vi "setSerializedData.vi"(0 "reference":refnum<class "CallEdge.lvclass">, 1 "startNode":refnum<class "AbstractNode.lvclass">, 2 "endNode":refnum<class "AbstractNode.lvclass">, 3 "xmlOut":string, 5 "error in (no error)":errorcluster) -> (14 "reference out":refnum<class "CallEdge.lvclass">, 19 "error out":errorcluster)   [LabVIEW 2014, in "CallEdge.lvclass"]
doc: "setSerializedData"
uses:
  <resource>/Framework/Providers/Open_GDS/UML/CallEdge_class/CallEdge.lvclass
  <resource>/Framework/Providers/Open_GDS/UML/AbstractNode_class/AbstractNode.lvclass
  <resource>/Framework/Providers/Open_GDS/UML/General/Point/Point Point2D.ctl
  <resource>/Framework/Providers/Open_GDS/UML/LineStyle_class/LineStyleType.ctl
  <resource>/Framework/Providers/Open_GDS/UML/ArrowHead_class/ArrowHeadType.ctl
  <resource>/Framework/Providers/Open_GDS/UML/LineStyle_class/LineStyle.lvclass
  <resource>/Framework/Providers/Open_GDS/UML/ArrowHead_class/ArrowHead.lvclass
  <resource>/Framework/Providers/Open_GDS/UML/SegmentedLineEdge_class/SegmentedLineEdge.lvclass
  <resource>/Framework/Providers/Open_GDS/UML/AbstractEdge_class/AbstractEdge.lvclass
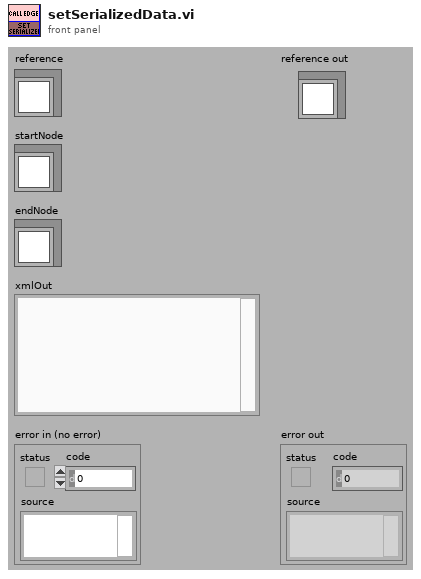
[diagram p1: front panel]
types:
  T1 = typedef "Point Point2D.ctl" = cluster{"x":dbl, "y":dbl}
  T2 = cluster{"Base class":cluster{"Base class":cluster{"Base class":cluster{"start":refnum<k1>, "end":refnum<k1>}}, "lineStyle":refnum<k1>, "startArrowHead":refnum<k1>, "endArrowHead":refnum<k1>, "startLabel":string, "midLabel":string, "endLabel":string, "MidLabelOffset":T1, "SplitWire":bool}, "signal":bool}
  T3 = typedef "LineStyle.lvclass/LineStyleType.ctl" = enum16{"SOLID", "DOTTED"}
  T4 = typedef "ArrowHead.lvclass/ArrowHeadType.ctl" = enum16{"NONE", "TRIANGLE", "BLACK_TRIANGLE", "V", "HALF_V", "DIAMOND", "BLACK_DIAMOND"}
  T5 = cluster{"Attributes":cluster{"Base class":cluster{"Base class":cluster{"Base class":cluster{"start":refnum<k1>, "end":refnum<k1>}}, "lineStyle":refnum<k1>, "startArrowHead":refnum<k1>, "endArrowHead":refnum<k1>, "startLabel":string, "midLabel":string, "endLabel":string, "MidLabelOffset":T1, "SplitWire":bool}, "signal":bool}, string, string, string}
  T6 = typedef "CallEdge.lvclass/ObjectAttributes.ctl" = cluster{"signal":bool}
  T7 = typedef "SegmentedLineEdge.lvclass/ObjectAttributes.ctl" = cluster{"lineStyle":refnum<class "LineStyle.lvclass">, "startArrowHead":refnum<class "ArrowHead.lvclass">, "endArrowHead":refnum<class "ArrowHead.lvclass">, "startLabel":string, "midLabel":string, "endLabel":string, "MidLabelOffset":T1, "SplitWire":bool}
  T8 = typedef "AbstractEdge.lvclass/ObjectAttributes.ctl" = cluster{"start":refnum<class "AbstractNode.lvclass">, "end":refnum<class "AbstractNode.lvclass">}
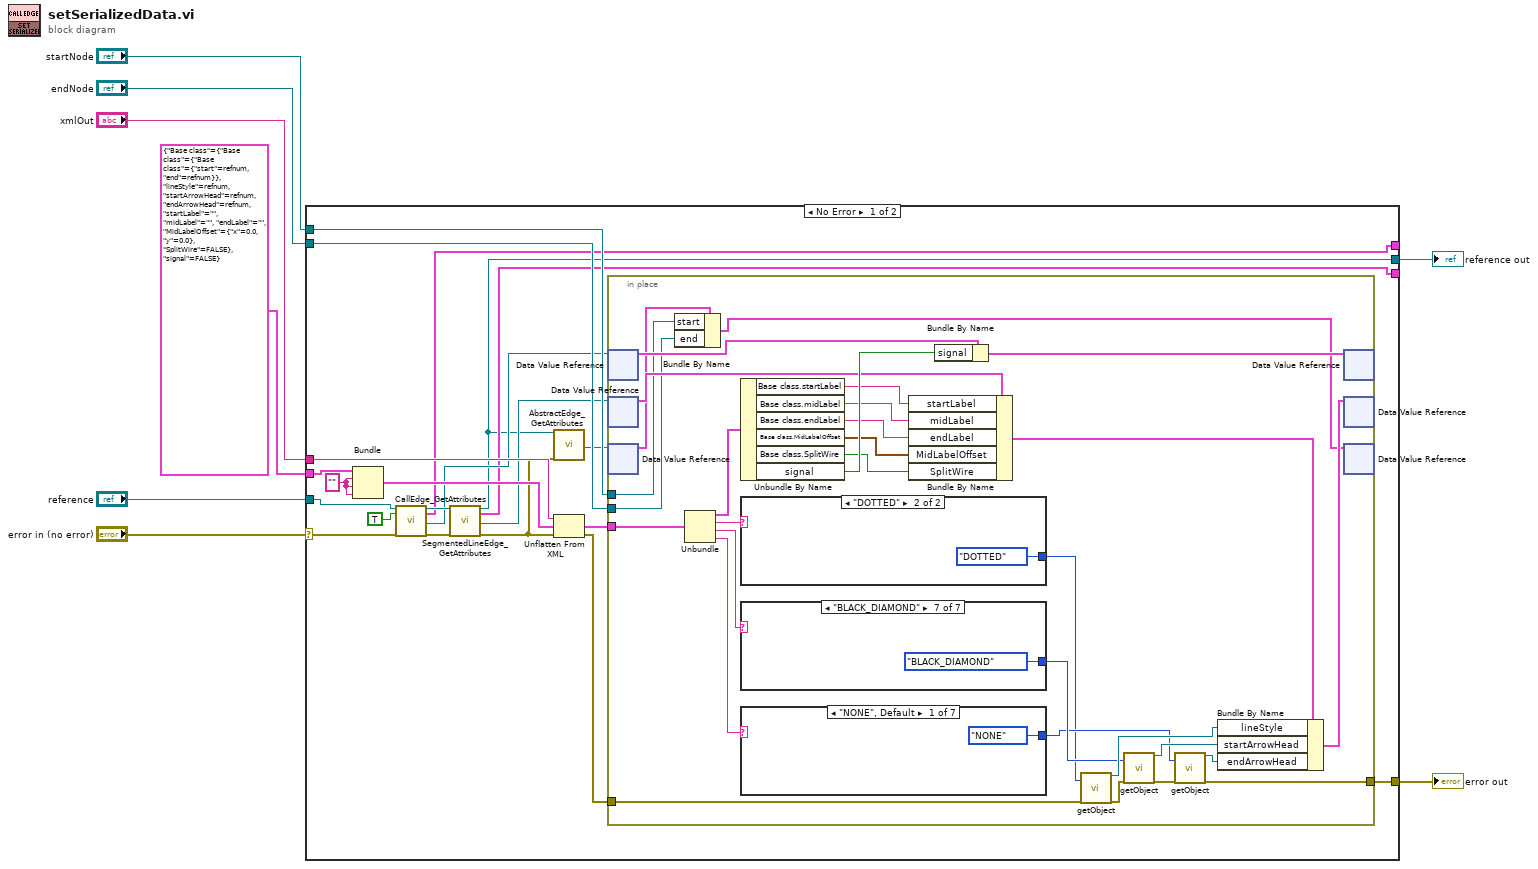
[diagram p0: block diagram]
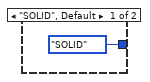
[diagram p2: hidden frame]
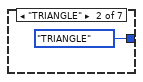
[diagram p3: hidden frame]
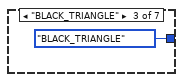
[diagram p4: hidden frame]
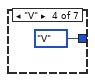
[diagram p5: hidden frame]
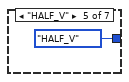
[diagram p6: hidden frame]
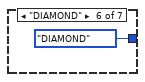
[diagram p7: hidden frame]
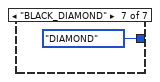
[diagram p8: hidden frame]
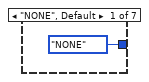
[diagram p9: hidden frame]
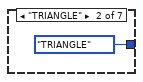
[diagram p10: hidden frame]
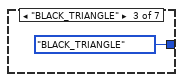
[diagram p11: hidden frame]
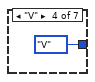
[diagram p12: hidden frame]
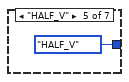
[diagram p13: hidden frame]
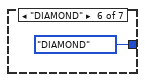
[diagram p14: hidden frame]
diagram:
  n1 = case shown="No Error" "error in (no error)" {
    selector: "error in (no error)" -> [w28 w76]
    tunnel: "reference" -> [w29 w77]
    tunnel: [w11 w77] -> w6
    tunnel: [w27 w76] -> w5
    tunnel: "xmlOut" -> [w18 _]
    tunnel: "startNode" -> [w26 _]
    tunnel: "endNode" -> [w25 _]
    tunnel: T2 {"Base class"={"Base class"={"Base class"={"start"=refnum, "end"=refnum}}, "lineStyle"=refnum, "startArrowHead"=refnum, "endArrowHead"=refnum, "startLabel"="", "midLabel"="", "endLabel"="", "MidLabelOffset"={"x"=0.0, "y"=0.0}, "SplitWire"=FALSE}, "signal"=FALSE} ("Attributes") -> [w23 _]
    tunnel: [w13 _] -> _
    tunnel: [w12 _] -> _
    frame No Error {
      w24 = ""
      n2 = Bundle("Attributes"=w23, w24, w24, w24) -> (w16:T5)  [unwired: 1 out]
      n3 = call <resource>:"CallEdge_GetAttributes.vi"("reference in"=w29, "OnlyGetDvrReference(False)"=TRUE, "error in (no error)"=w28) -> ("reference out"=w21:refnum<class "CallEdge.lvclass">, "Data"=w13:T6, "DataRef"=w15:refnum<data-value>, "error out"=w20:errorcluster)  [unwired: 13 in]
      n4 = call <resource>:"SegmentedLineEdge_GetAttributes.vi"("reference in"=w21, "error in (no error)"=w20) -> ("reference out"=w11:refnum<class "CallEdge.lvclass">, "Data"=w12:T7, "DataRef"=w14:refnum<data-value>, "error out"=w10:errorcluster)  [unwired: 14 in]
      n5 = call <resource>:"AbstractEdge_GetAttributes.vi"("reference in"=w11, "error in (no error)"=w10) -> ("DataRef"=w9:refnum<data-value>)  [unwired: 14 in, 3 out]
      n6 = Unflatten From XML(xml string=w18, type=w16, error in (no error)=w10) -> (value=w19:T5, error out=w17:errorcluster)
      n7 = in-place {
        in-place-border: [w54] -> w27
        in-place-border: w26 -> [w38]
        in-place-border: w25 -> [w37]
        in-place-border: w19 -> [w50]
        in-place-border: w17 -> [w49]
        n8 = in-place-dvr #1(w15) -> (w41:T6)  [unwired: 1 out]
        n9 = in-place-dvr #2(w14) -> (w39:T7)  [unwired: 1 out]
        n10 = in-place-dvr #3(w9) -> (w34:T8)  [unwired: 1 out]
        n11 = Bundle By Name(cluster=w34, "start"=w38, "end"=w37) -> (w33:T8)
        n12 = Unbundle(w50) -> ("Attributes"=w42:T2, w32:string, w31:string, w30:string)
        n13 = Unbundle By Name(w42) -> ("Base class.startLabel"=w43:string, "Base class.midLabel"=w44:string, "Base class.endLabel"=w45:string, "Base class.MidLabelOffset"=w46:T1, "Base class.SplitWire"=w47:bool, "signal"=w48:bool)
        n14 = case shown="\"DOTTED\"" w32 {
          tunnel: [LineStyleType."SOLID" ("lineStyle") LineStyleType."DOTTED" ("lineStyle")] -> w51
          frame "SOLID", Default {
          }
          frame "DOTTED" {
          }
        }
        n15 = case shown="\"BLACK_DIAMOND\"" w31 {
          tunnel: [ArrowHeadType."NONE" ("arrowHead") ArrowHeadType."TRIANGLE" ("arrowHead") ArrowHeadType."BLACK_TRIANGLE" ("arrowHead") ArrowHeadType."V" ("arrowHead") ArrowHeadType."HALF_V" ("arrowHead") ArrowHeadType."DIAMOND" ("arrowHead") ArrowHeadType."BLACK_DIAMOND" ("arrowHead")] -> w53
          frame "NONE", Default {
          }
          frame "TRIANGLE" {
          }
          frame "BLACK_TRIANGLE" {
          }
          frame "V" {
          }
          frame "HALF_V" {
          }
          frame "DIAMOND" {
          }
          frame "BLACK_DIAMOND" {
          }
        }
        n16 = case shown="\"NONE\", Default" w30 {
          tunnel: [ArrowHeadType."NONE" ("arrowHead") ArrowHeadType."TRIANGLE" ("arrowHead") ArrowHeadType."BLACK_TRIANGLE" ("arrowHead") ArrowHeadType."V" ("arrowHead") ArrowHeadType."HALF_V" ("arrowHead") ArrowHeadType."DIAMOND" ("arrowHead") ArrowHeadType."DIAMOND" ("arrowHead")] -> w52
          frame "NONE", Default {
          }
          frame "TRIANGLE" {
          }
          frame "BLACK_TRIANGLE" {
          }
          frame "V" {
          }
          frame "HALF_V" {
          }
          frame "DIAMOND" {
          }
          frame "BLACK_DIAMOND" {
          }
        }
        n17 = Bundle By Name(cluster=w39, "startLabel"=w43, "midLabel"=w44, "endLabel"=w45, "MidLabelOffset"=w46, "SplitWire"=w47) -> (w36:T7)
        n18 = Bundle By Name(cluster=w41, "signal"=w48) -> (w40:T6)
        n19 = call <resource>:"getObject.vi"("lineStyle"=w51, "error in (no error)"=w49) -> ("reference out"=w59:refnum<class "LineStyle.lvclass">, "error out"=w58:errorcluster)  [unwired: 16 out]
        n20 = call <resource>:"getObject.vi"("arrowHead"=w53, "error in (no error)"=w58) -> ("reference out"=w55:refnum<class "ArrowHead.lvclass">, "error out"=w57:errorcluster)  [unwired: 16 out]
        n21 = call <resource>:"getObject.vi"("arrowHead"=w52, "error in (no error)"=w57) -> ("reference out"=w56:refnum<class "ArrowHead.lvclass">, "error out"=w54:errorcluster)  [unwired: 16 out]
        n22 = Bundle By Name(cluster=w36, "lineStyle"=w59, "startArrowHead"=w55, "endArrowHead"=w56) -> (w35:T7)
        n23 = in-place-dvr #1(w40) -> ()  [unwired: 2 out]
        n24 = in-place-dvr #2(w35) -> ()  [unwired: 2 out]
        n25 = in-place-dvr #3(w33) -> ()  [unwired: 2 out]
      }
    }
    frame Error {
    }
  }
  "reference out" <- w6
  "error out" <- w5
